vi "Mean plot, Statistics.vi"(6 "Gene Name":string, 7 "배열":dbl[][](array[numeric])) -> (1 "Reject null hypothesis":bool, 2 "P-value":dbl, 3 "Plot":cluster{i32[], "배열":dbl[]}[](graph) caption="Fos")   [LabVIEW 2017]
uses:
  <vilib>/Analysis/NI_AALBase.lvlib
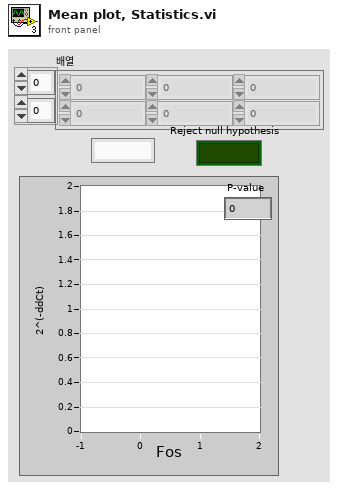
[diagram p1: front panel]
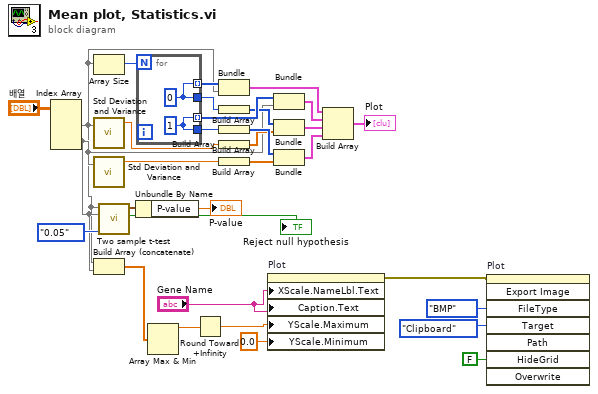
[diagram p0: block diagram]
diagram:
  n1 = Index Array(array="배열") -> (element #1=w7:dbl[], element #2=w8:dbl[])  [unwired: 4 in]
  n2 = Array Size(array=w7) -> (size(s)=w31:i32)
  n3 = call <vilib>:"Std Deviation and Variance.vi"("X"=w7) -> ("mean"=w19:dbl)  [unwired: 1 in, 2 out]
  n4 = call <vilib>:"Std Deviation and Variance.vi"("X"=w8) -> ("mean"=w21:dbl)  [unwired: 1 in, 2 out]
  n5 = Build Array (concatenate)(w7, w8) -> (w6:dbl[])
  n6 = call "Two sample t-test.vi"("Significant level"=enum16{"0.05", "0.01"}."0.05", "Data SET II"=w8, "Data SET I"=w7) -> ("Reject null hypothesis"=→"Reject null hypothesis":bool, "t-Test Statistics"=w14:cluster{"t-Value":dbl, "DF":i32, "P-value":dbl})  [unwired: 3 in]
  n7 = Unbundle By Name(w14) -> ("P-value"=→"P-value":dbl)
  n8 = for {
    N: w31 -> [_]
    tunnel: [w33] -> w30 mode=indexing
    tunnel: [w34] -> w29 mode=indexing
    tunnel: [w34] -> w25
    tunnel: [w33] -> w23
    w34 = 1
    w33 = 0
  }
  n9 = Array Max & Min(array=w6) -> (max value=w10:dbl)  [unwired: 3 out]
  n10 = Round Toward +Infinity(x=w10) -> (ceil(x): smallest int >= x=w9:dbl)
  n11 = Bundle(w30, "배열"=w7) -> (w28:cluster{i32[], "배열":dbl[]})  [unwired: 1 in]
  n12 = Build Array(w23) -> (w22:i32[])
  n13 = Build Array(w25) -> (w24:i32[])
  n14 = Build Array(w19) -> (w18:dbl[])
  n15 = Build Array(w21) -> (w20:dbl[])
  n16 = property on="Plot" class="XYGraph (strict)"("XScale.NameLbl.Text"="Gene Name", "Caption.Text"="Gene Name", "YScale.Maximum"=w9, "YScale.Minimum"=0.0 ("Y 스케일.범위:최소값")) -> (error out=w4:errorcluster)  [unwired: 2 in, 1 out]
  n17 = Bundle(w29, "배열"=w8) -> (w27:cluster{i32[], "배열":dbl[]})  [unwired: 1 in]
  n18 = Bundle(w22, w18) -> (w17:cluster{i32[], dbl[]})  [unwired: 1 in]
  n19 = Bundle(w24, w20) -> (w16:cluster{i32[], dbl[]})  [unwired: 1 in]
  n20 = Build Array(w28, w27, w17, w16) -> (→"Plot":cluster{i32[], "배열":dbl[]}[])
  n21 = invoke on="Plot" class="XYGraph (엄격한)" method="Export Image"(error in=w4, "FileType"=enum32{"BMP", "EPS", "EMF", "PICT"}."BMP" ("파일 타입"), "Target"=enum32{"File", "Clipboard"}."Clipboard" ("타겟"), "HideGrid"=FALSE ("눈금 숨기기")) -> ()  [unwired: 4 in, 8 out]
